vi "pulse creation.vi"(7 "DAQmx Task Name":refnum<k21>="chop2", 8 "error in":errorcluster, 10 "task/channels in":refnum<k21>="testcurrent", 11 "chopper width(usec)":u32=400) -> (0 "error out":errorcluster, 1 "std percent":dbl format="%0.2f", 2 "mean":dbl format="%0.2f", 3 "Waveform Graph 2":dbl[](graph), 4 "standard deviation":dbl format="%0.2f")   [LabVIEW 2016]
doc: "Sends a pulse to the chopper. Then the stable current is measured in the offset cup"
uses:
  <vilib>/DAQmx/write.llb/DAQmx Write (Digital Wfm 1Chan NSamp).vi
  <vilib>/DAQmx/read.llb/DAQmx Read (Analog 1D DBL 1Chan NSamp).vi
  <vilib>/DAQmx/miscellaneous.llb/DAQmx Fill In Error Info.vi
  <vilib>/Waveform/DWDTOps.llb/DWDT Uncompress Digital.vi
  <resource>/objmgr/daqmx.rc
  <vilib>/Analysis/NI_AALBase.lvlib
panel:
  out "min index(es)":i32
  out "max index(es)":i32
  out "min value":dbl
  out "max value":dbl
  out "error out 4":errorcluster
  in  "stop":bool
  out "subarray 3":dbl[](array[numeric])
  out "error out 3":errorcluster
  out "sum":dbl
  out "stop? 2":bool
  out "stop?":bool
  out "error out 2":errorcluster
  out "error out 6":errorcluster
  out "error out 5":errorcluster
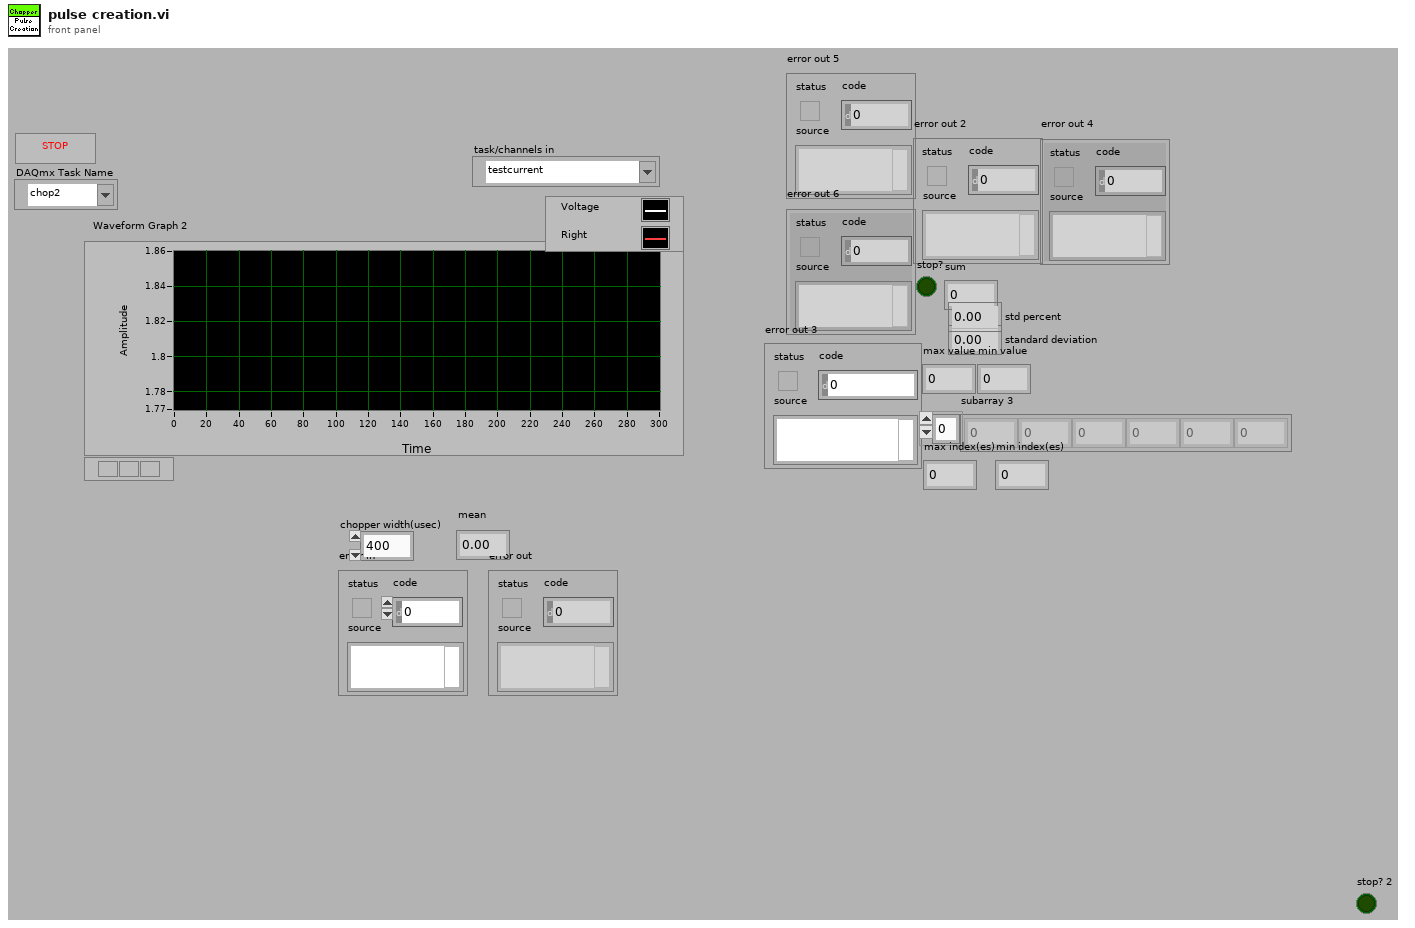
[diagram p1: front panel]
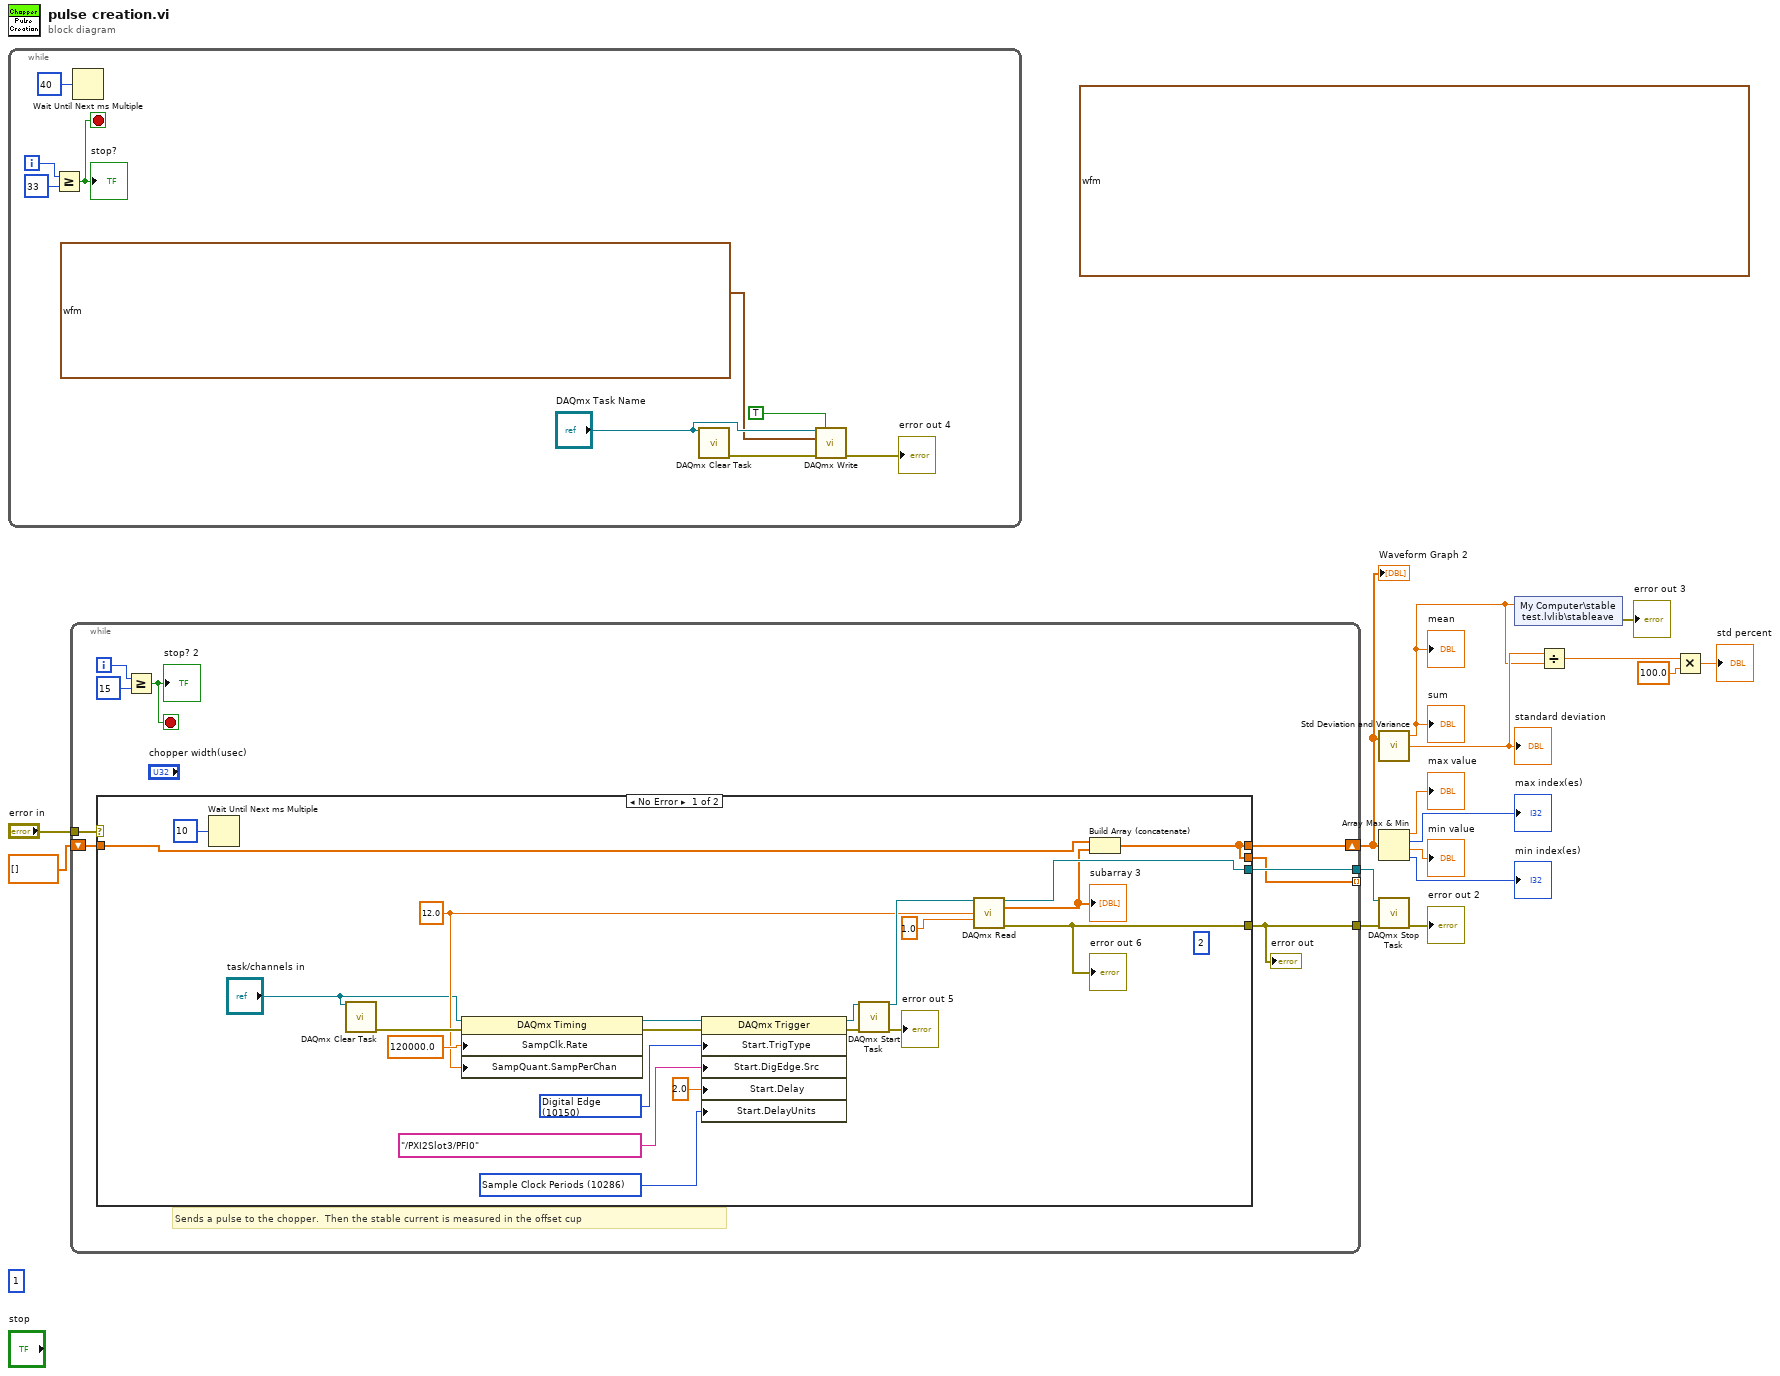
[diagram p0: block diagram]
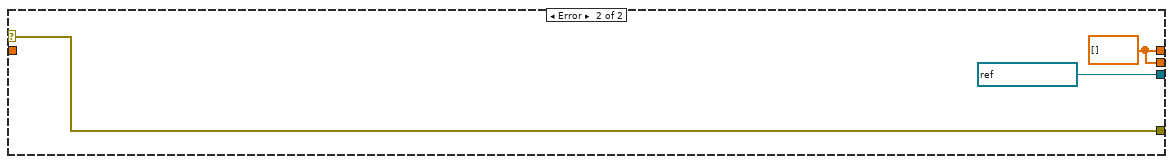
[diagram p2: hidden frame]
diagram:
  (unwired) digitalwaveform {"t0"=timestamp(0 s since 1904-01-01), "dt"=0.0001, "Y"={"transitions"=[], "data"=array1150x16[18400 elements]}} ("digital waveform")
  (unwired) 1 ("index")
  n1 = while {
    i -> [w22]
    stop <- w20 stop-if-true
    n2 = Greater Or Equal?(x=w22, y=33) -> (x >= y?=w20:bool)
    "stop?" <- w20
    n3 = Wait Until Next ms Multiple(millisecond multiple=u32 40) -> ()  [unwired: 1 out]
    n4 = call <vilib>:"DAQmx Clear Task.vi"("task in"="DAQmx Task Name") -> ("error out"=w25:errorcluster)  [unwired: 14 in]
    n5 = call-poly <vilib>:"DAQmx Write.vi"("task/channels in"="DAQmx Task Name", "auto start"=TRUE, "data"=digitalwaveform {"t0"=timestamp(0 s since 1904-01-01), "dt"=0.0001, "Y"={"transitions"=[], "data"=array1150x16[18400 elements]}} ("digital waveform"), "error in"=w25) -> ("error out"=→"error out 4":errorcluster)  [unwired: 9 in, 2 out]
  }
  n6 = while {
    tunnel: "error in" -> [w34]
    tunnel: [w33] -> w15
    tunnel: [w32] -> w14
    shift-right: [w31] -> w1
    shift-left: dbl[] [] -> [w30]
    tunnel: [w26] -> _ mode=indexing
    i -> [w28]
    stop <- w29 stop-if-true
    # "Sends a pulse to the chopper.  Then the stable current is measured in the offset cup"
    n7 = case shown="No Error" w34 {
      selector: w34 -> [_ w58]
      tunnel: [w48 w58] -> w32
      tunnel: [w49 refnum<k21> "testcurrent" ("task out")] -> w33
      tunnel: [w39 w56] -> w31
      tunnel: w30 -> [w47 _]
      tunnel: [w39 w56] -> w26
      frame No Error {
        w38 = 10286 items=["Sample Clock Periods"=10286, "Seconds"=10364, "Ticks"=10304] ("Start.DelayUnits")
        w50 = 10150 items=["Analog Edge"=10099, "Digital Edge"=10150, "Digital Pattern"=10398, "Analog Window"=10103, "None"=10230] ("Start.TrigType")
        (unwired) 2 ("index (row)")
        w41 = 12.0 ("SampClk.Rate")
        n8 = Wait Until Next ms Multiple(millisecond multiple=u32 10) -> ()  [unwired: 1 out]
        n9 = call <vilib>:"DAQmx Clear Task.vi"("task in"="task/channels in") -> ("error out"=w45:errorcluster)  [unwired: 14 in]
        n10 = property class="DAQmx Timing"(reference="task/channels in", error in=w45, "SampClk.Rate"=120000.0, "SampQuant.SampPerChan"=w41) -> (reference out=w46:refnum<k21>, error out=w43:errorcluster)
        n11 = property class="DAQmx Trigger"(reference=w46, error in=w43, "Start.TrigType"=w50, "Start.DigEdge.Src"=tag "/PXI2Slot3/PFI0", "Start.Delay"=2.0, "Start.DelayUnits"=w38) -> (reference out=w44:refnum<k21>, error out=w42:errorcluster)
        n12 = call <vilib>:"DAQmx Start Task.vi"("task/channels in"=w44, "error in"=w42) -> ("task out"=w55:refnum<k21>, "error out"=→"error out 5":errorcluster)  [unwired: 12 in]
        n13 = call-poly <vilib>:"DAQmx Read.vi"("task/channels in"=w55, "number of samples per channel"=w41, "timeout"=1.0) -> ("task out"=w49:refnum<k21>, "data"=w40:dbl[], "error out"=w48:errorcluster)  [unwired: 10 in]
        "error out 6" <- w48
        "subarray 3" <- w40
        n14 = Build Array (concatenate)(w47, w40) -> (w39:dbl[])
      }
      frame Error {
        w56 = dbl[] []
      }
    }
    "error out" <- w32
    n15 = Greater Or Equal?(x=w28, y=15) -> (x >= y?=w29:bool)
    "stop? 2" <- w29
  }
  "Waveform Graph 2" <- w1
  n16 = call <vilib>:"Std Deviation and Variance.vi"("X"=w1) -> ("mean"=w9:dbl, "standard deviation"=w10:dbl)  [unwired: 1 in, 1 out]
  "sum" <- w9
  "mean" <- w9
  "standard deviation" <- w10
  n17 = Array Max & Min(array=w1) -> (max value=→"max value":dbl, max index (indices)=→"max index(es)":i32, min value=→"min value":dbl, min index (indices)=→"min index(es)":i32)
  n18 = call <vilib>:"DAQmx Stop Task.vi"("task/channels in"=w15, "error in"=w14) -> ("error out"=→"error out 2":errorcluster)  [unwired: 12 in, 1 out]
  n19 = shared-variable "My Computer\\stable test.lvlib\\stableave"(w9) -> (error out=→"error out 3":errorcluster)  [unwired: 1 in]
  n20 = Divide(x=w10, y=w9) -> (x/y=w8:dbl)
  n21 = Multiply(x=w8, y=100.0) -> (x*y=→"std percent":dbl)
